vi "Init.vi"(8 "error in (no error)":errorcluster, 11 "uService Template in":refnum<class "DAQ Manager.lvclass">) -> (0 "error out":errorcluster, 3 "uService Template out":refnum<class "DAQ Manager.lvclass">)   [LabVIEW 2020, in "DAQ Manager.lvlib" / "DAQ Manager.lvclass"]
uses:
  DAQ Manager.lvclass
  Interfaces/DAQ Control/DAQ Control.lvclass
  Ancestor/Ancestor/Ancestor.lvclass/Ancestor.ctl
  DAQ Manager.lvclass/DAQ Manager.ctl
  Support VIs/Generate Error.vi
  FGV/Error Memory/Get Error Description.vi
  Support VIs/Get PC name.vi
  Ancestor/Ancestor/Read ID.vi
  Support VIs/Get Class Name.vi
  <vilib>/Utility/error.llb/Clear Errors.vi
  FGV/Error Memory/Error Memory Core.vi
  <vilib>/AdvancedString/Delimited String to 1D String Array.vi
  Support VIs/Circus Root Path.vi
  FGV/Error Memory/Error Crt Lvl checker.vi
  FGV/Error Memory/Error Memory Core.vi/40c8088d-b597-4017-91af-faa98e00292e.vi
  FGV/Error Memory/Error Memory Core.vi/d4a3ab98-063c-4e44-b43d-fbdcfe6c2be2.vi
  Support VIs/Global Memory.vi
  <vilib>/Utility/LVClass/Get LV Class Name.vi
  Support VIs/Is in Packed Library.vi
  Support VIs/TALOS Root path.vi
  Support VIs/Read CSV worksheet.vi
  Support VIs/Global Constants.vi
  <vilib>/Utility/error.llb/General Error Handler.vi
  <vilib>/Utility/config.llb/Open Config Data.vi
  <vilib>/Utility/config.llb/Get Section Names.vi
  <vilib>/Utility/config.llb/Get Key Names.vi
  <vilib>/Utility/config.llb/Read Key.vi
  <vilib>/Utility/config.llb/Read Key (String).vi
  <vilib>/Utility/config.llb/Close Config Data.vi
  <vilib>/Utility/error.llb/Search and Replace Pattern.vi
  Support VIs/Error Log.vi
  Ancestor/Ancestor/Ancestor.lvclass
  <vilib>/Comparison/Equal/Equal Functor/Equal Functor.lvclass
  TALOS.lvlib
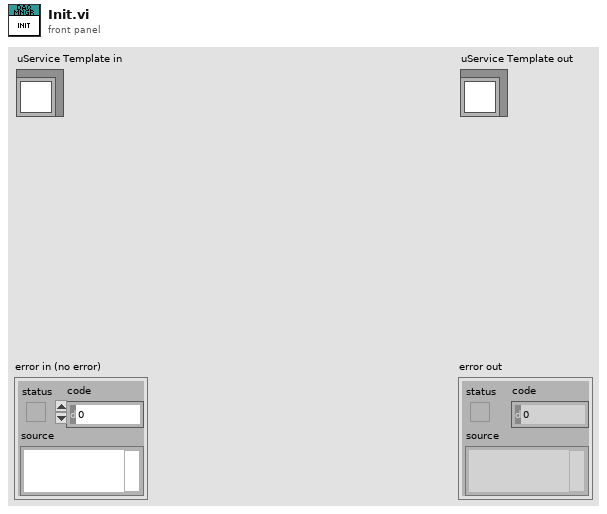
[diagram p1: front panel]
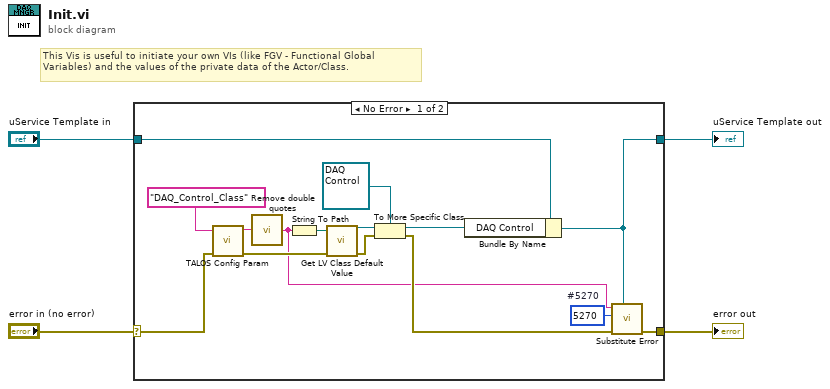
[diagram p0: block diagram]
diagram:
  # "This Vis is useful to initiate your own VIs (like FGV - Functional Global Variables) and the values of the private data of the Actor/Class."
  n1 = case shown="No Error" "error in (no error)" {
    selector: "error in (no error)" -> [w5 w20]
    tunnel: "uService Template in" -> [w18 w21]
    tunnel: [w10 w21] -> w4
    tunnel: [w8 w20] -> w3
    frame No Error {
      w13 = 5270  # #5270
      n2 = call "TALOS Config Param.vi"("error in (no error)"=w5, "Parameter Name"="DAQ_Control_Class") -> ("error out"=w19:errorcluster, "Output"=w6:string)  [unwired: 8 in]
      n3 = call "Remove double quotes.vi"("Input string"=w6) -> ("Output string"=w9:string)  [unwired: 4 in]
      n4 = String To Path(string=w9) -> (path=w17:path)
      n5 = call <vilib>:"Get LV Class Default Value.vi"("error in (no error)"=w19, "class path"=w17) -> ("error out"=w16:errorcluster, "object"=w15:refnum<class>)  [unwired: 8 in]
      n6 = To More Specific Class(target class=refnum<class "DAQ Control.lvclass"> refnum ("DAQ Control Interface"), reference=w15, error in=w16) -> (specific class reference=w11:refnum<class "DAQ Control.lvclass">, error out=w14:errorcluster)
      n7 = Bundle By Name(cluster=w18, "DAQ Control"=w11) -> (w10:refnum<class "DAQ Manager.lvclass">)
      n8 = call "Substitute Error.vi"("LabVIEW Object"=w10, "error in (no error)"=w14, "Error Code"=w13, "Optional String"=w9) -> ("error out"=w8:errorcluster)  [unwired: 7 in]
    }
    frame Error {
    }
  }
  "error out" <- w3
  "uService Template out" <- w4
